vi "Omron TCP FINS-Request And Respond.vi"(8 "error in":errorcluster, 11 "Buffer Data In":T1) -> (0 "error out":errorcluster, 3 "Buffer Data Out":T1)   [LabVIEW 2016]
uses:
  Data Def/Omron TCP FINS-Buffer Data.ctl
  Data Def/Omron TCP FINS-Command Code.ctl
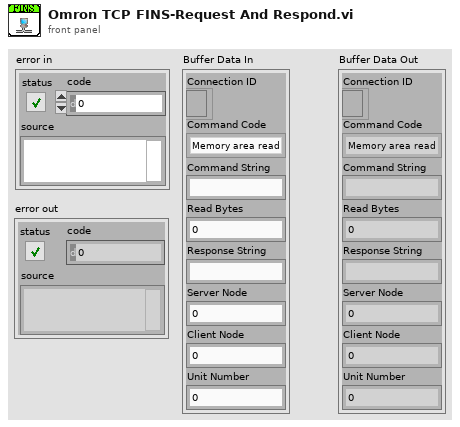
[diagram p1: front panel]
types:
  T1 = typedef "Omron TCP FINS-Buffer Data.ctl" = cluster{"Connection ID":refnum<k5>, "Command Code":T2, "Command String":string, "Read Bytes":i32, "Response String":string, "Server Node":u8, "Client Node":u8, "Unit Number":u8}
  T2 = typedef "Omron TCP FINS-Command Code.ctl" = enum16{"Memory area read", "Memory area write"}
  T3 = enum16{"Standard", "Buffered", "CRLF", "Immediate"}
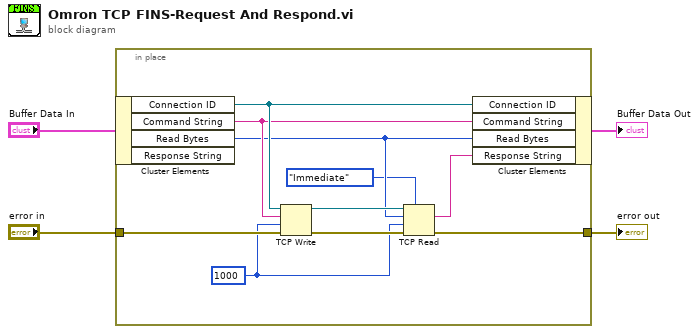
[diagram p0: block diagram]
diagram:
  n1 = in-place {
    in-place-border: "error in" -> [w14]
    in-place-border: [w9] -> w1
    w8 = 1000 ("timeout ms (25000)")
    n2 = in-place-cluster #1("Buffer Data In") -> ("Connection ID"=w13:refnum<k5>, "Command String"=w12:string, "Read Bytes"=w7:i32)  [unwired: 1 out]
    n3 = TCP Write(connection ID=w13, data in=w12, error in (no error)=w14, 9:w8) -> (connection ID out=w11:refnum<k5>, error out=w10:errorcluster)  [unwired: 1 out]
    n4 = TCP Read(connection ID=w11, bytes to read=w7, error in (no error)=w10, 7:T3."Immediate" ("mode (standard)"), 9:w8) -> (data out=w6:string, error out=w9:errorcluster)  [unwired: 1 out]
    n5 = in-place-cluster #1("Connection ID"=w13, "Command String"=w12, "Read Bytes"=w7, "Response String"=w6) -> (→"Buffer Data Out":T1)
  }
  "error out" <- w1
